vi "xy graph.vi"() -> ()   [LabVIEW 2014]
doc: "Es VI te permite explorar de manera basica lo socntroles e indicadores de un programa en Labview."
panel:
  out "XY Graph":cluster{"Y":dbl[], "Y":dbl[]}[](graph)
  in  "stop":bool
  # "XY Graph"
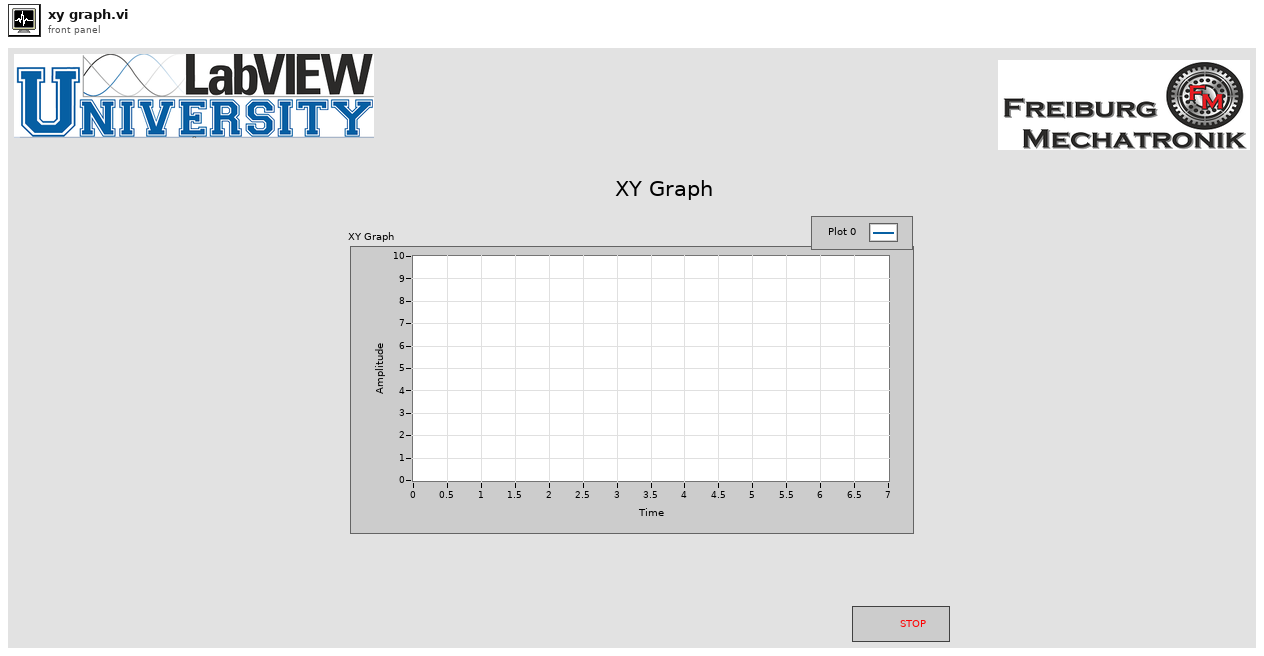
[diagram p1: front panel]
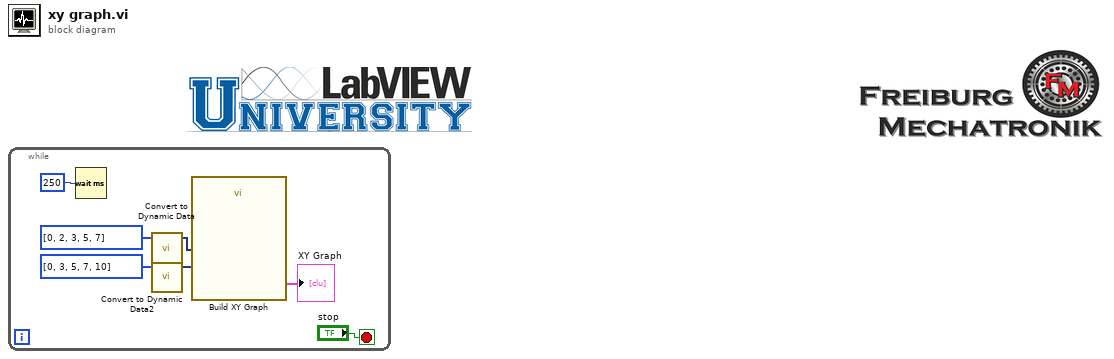
[diagram p0: block diagram]
diagram:
  n1 = while {
    stop <- "stop" stop-if-true
    n2 = Wait (ms)(milliseconds to wait=u32 250) -> ()  [unwired: 1 out]
    n3 = call "Convert to Dynamic Data"("Array"=i32[] [0, 2, 3, 5, 7]) -> ("Dynamic Data Type"=w4:dynamicdata)  [unwired: 3 in]
    n4 = call "Convert to Dynamic Data2"("Array"=i32[] [0, 3, 5, 7, 10]) -> ("Dynamic Data Type"=w3:dynamicdata)  [unwired: 3 in]
    n5 = call "Build XY Graph"("Y Input"=w3, "X Input"=w4) -> ("XY Graph"=→"XY Graph":cluster{"Y":dbl[], "Y":dbl[]}[])  [unwired: 3 in, 6 out]
  }
